vi "Train Tip KNN.vi"(8 "error in (no error)":errorcluster, 9 "Classifier File":path=path "C:/Users/Andrew/Documents/Apatite to Zircon Code/Track Finding/TipClassifier.knn", 10 "Non-tip Data File":path=path "C:/Users/Andrew/Documents/Apatite to Zircon Code/Track Finding/Non-tip Data.csv", 11 "Tip Data File":path=path "C:/Users/Andrew/Documents/Apatite to Zircon Code/Track Finding/Tip Data.csv") -> (0 "error out":errorcluster, 1 "Class Predictive Value":dbl[](array[numeric]) format="%.2f", 2 "Classification Distribution":i32[][](array[numeric]), 3 "Accuracy":sgl format="%.2f")   [LabVIEW 2013]
uses:
  <vilib>/vision/Classification.llb/IMAQ Classifier Nearest Neighbor options.ctl
  <vilib>/Utility/file.llb/Read From Spreadsheet File (DBL).vi
  <vilib>/vision/NI_Vision_Development_Module.lvlib
panel:
  in  "Nearest Neighbor Options":T1={"Method"=1, "Metric"=2, "k"=4} {"Method" items=["Nearest Neighbor", "K Nearest Neighbor", "Minimum Mean Distance"]; "Metric" items=["Maximum", "Sum", "Euclidean"]; "k" min=3}
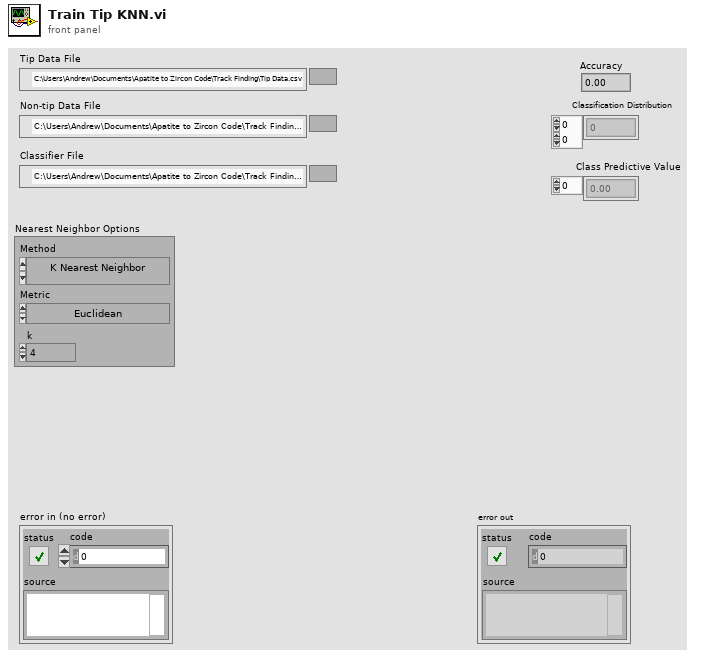
[diagram p1: front panel]
types:
  T1 = typedef "IMAQ Classifier Nearest Neighbor options.ctl" = cluster{"Method":i32, "Metric":i32, "k":i32}
  T2 = typedef "Image Type" = u32
  T3 = typedef "IMAQ Image.ctl" = refnum<image>
  T4 = typedef "IMAQ Classifier Session.ctl" = refnum<k1>
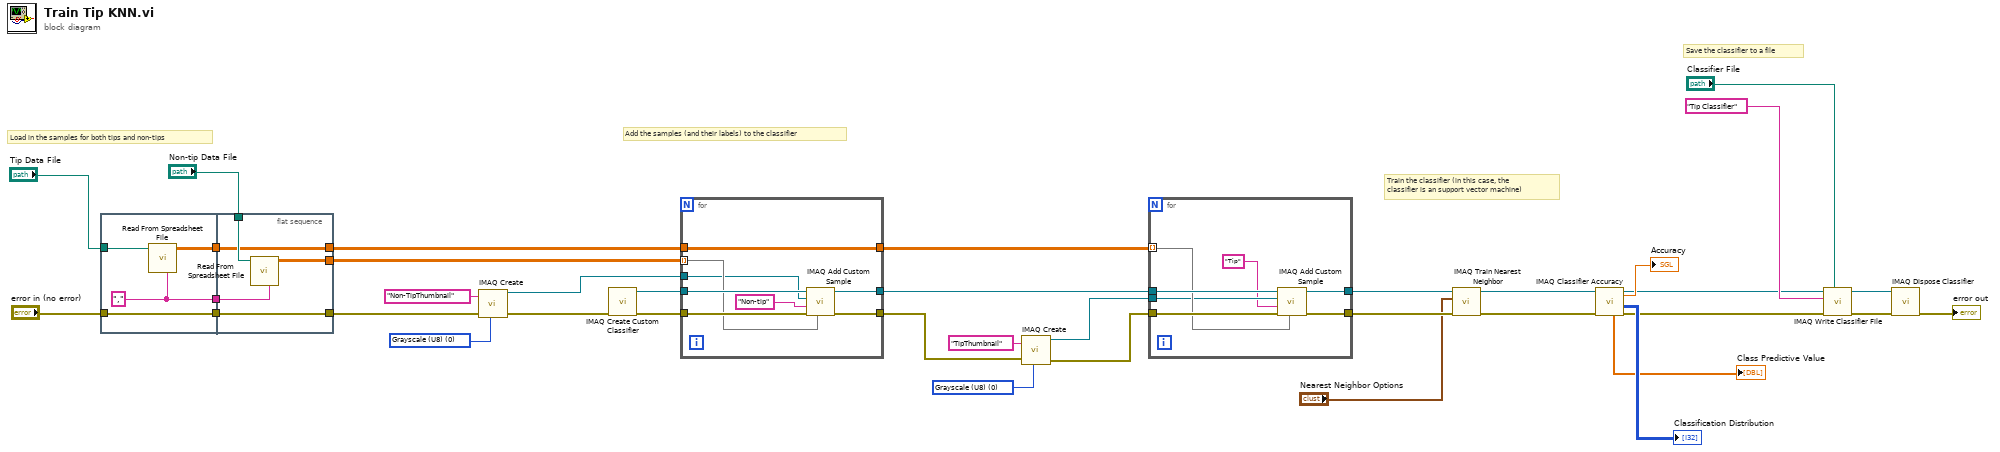
[diagram p0: block diagram]
diagram:
  w26 = T2 0 items=["Grayscale (U8)", "Grayscale (I16)", "Grayscale (SGL)", "Complex (CSG)", "RGB (U32)", "HSL (U32)", "RGB (U64)", "Grayscale (U16)"] ("Image Type")
  w28 = T2 0 items=["Grayscale (U8)", "Grayscale (I16)", "Grayscale (SGL)", "Complex (CSG)", "RGB (U32)", "HSL (U32)", "RGB (U64)", "Grayscale (U16)"] ("Image Type")
  # "Save the classifier to a file"
  # "Train the classifier (in this case, the \nclassifier is an support vector machine)"
  # "Add the samples (and their labels) to the classifier"
  # "Load in the samples for both tips and non-tips"
  n1 = flat-sequence {
    tunnel: "Tip Data File" -> [w41]
    tunnel: "error in (no error)" -> [w40]
    tunnel: [w40] -> w35
    tunnel: [w39] -> w33
    tunnel: [w38] -> w21
    tunnel: [w46] -> w24
    tunnel: w35 -> [w46]
    tunnel: "Non-tip Data File" -> [w45]
    tunnel: [w44] -> w19
    tunnel: w33 -> [w43]
    tunnel: [w43] -> w20
    tunnel: w21 -> [w42]
    frame #0 {
      w38 = "," ("delimiter (\\t)")
      n2 = call-poly <vilib>:"Read From Spreadsheet File.vi"("delimiter (\\t)"=w38, "file path (dialog if empty)"=w41) -> ("all rows"=w39:dbl[][])  [unwired: 5 in, 4 out]
    }
    frame #1 {
      n3 = call-poly <vilib>:"Read From Spreadsheet File.vi"("delimiter (\\t)"=w42, "file path (dialog if empty)"=w45) -> ("all rows"=w44:dbl[][])  [unwired: 5 in, 4 out]
    }
  }
  n4 = call "IMAQ Create"("Image Name"="Non-TipThumbnail", "Image Type"=w26, "error in (no error)"=w24) -> ("New Image"=w18:T3, "error out"=w17:errorcluster)  [unwired: 2 in]
  n5 = call "IMAQ Create Custom Classifier"("error in (no error)"=w17) -> ("error out"=w31:errorcluster, "Classifier Session"=w32:T4)  [unwired: 9 in]
  n6 = for {
    tunnel: w19 -> [w52] mode=indexing
    tunnel: w32 -> [w53]
    tunnel: w31 -> [w54]
    tunnel: [w51] -> w29
    tunnel: [w50] -> w23
    tunnel: w20 -> [w49]
    tunnel: [w49] -> w30
    tunnel: w18 -> [w47]
    n7 = call "IMAQ Add Custom Sample"("Feature Vector"=w52, "error in (no error)"=w54, "Class"="Non-tip", "Image"=w47, "Classifier Session"=w53) -> ("error out"=w50:errorcluster, "Classifier Session (dup)"=w51:T4)  [unwired: 5 in]
  }
  n8 = call "IMAQ Create"("Image Name"="TipThumbnail", "Image Type"=w28, "error in (no error)"=w23) -> ("New Image"=w16:T3, "error out"=w15:errorcluster)  [unwired: 2 in]
  n9 = for {
    tunnel: w30 -> [w59] mode=indexing
    tunnel: w29 -> [w60]
    tunnel: w15 -> [w61]
    tunnel: [w58] -> w10
    tunnel: [w57] -> w9
    tunnel: w16 -> [w56]
    n10 = call "IMAQ Add Custom Sample"("Feature Vector"=w59, "error in (no error)"=w61, "Class"="Tip", "Image"=w56, "Classifier Session"=w60) -> ("error out"=w57:errorcluster, "Classifier Session (dup)"=w58:T4)  [unwired: 5 in]
  }
  n11 = call "IMAQ Train Nearest Neighbor"("error in (no error)"=w9, "Nearest Neighbor Options"="Nearest Neighbor Options", "Classifier Session"=w10) -> ("error out"=w4:errorcluster, "Classifier Session (dup)"=w5:T4)  [unwired: 5 in, 2 out]
  n12 = call "IMAQ Classifier Accuracy"("error in (no error)"=w4, "Classifier Session"=w5) -> ("error out"=w2:errorcluster, "Classification Distribution"=→"Classification Distribution":i32[][], "Classifier Session (dup)"=w3:T4, "Class Predictive Value"=→"Class Predictive Value":dbl[], "Accuracy"=→"Accuracy":sgl)  [unwired: 3 in, 2 out]
  n13 = call "IMAQ Write Classifier File"("File Path"="Classifier File", "error in (no error)"=w2, "Description"="Tip Classifier", "Classifier Session"=w3) -> ("error out"=w14:errorcluster, "Classifier Session (dup)"=w13:T4)  [unwired: 6 in]
  n14 = call "IMAQ Dispose Classifier"("error in (no error)"=w14, "Classifier Session"=w13) -> ("error out"=→"error out":errorcluster)  [unwired: 9 in]
